vi "Impulse Response Function.vi"(1 "Signal Y Response":dbl[](array[numeric]) format="%0.2f", 2 "Signal X Stimulus":dbl[](array[numeric]) format="%0.2f") -> (0 "Impulse Response":dbl[](array[numeric]) format="%0.2f")   [LabVIEW 2020, in "NI_AALPro.lvlib"]
doc: "Computes the impulse response of a network based on time-domain signals Signal X Stimulus and Signal Y Response. The impulse response is in the time domain, so you do not need to convert time units to frequency units. The impulse response is the inverse transform of the transfer function.\n\nThe VI computes Impulse Response as\n Inverse Real FFT [ Sxy(f) / Sxx(f) ]\n\nSignal X Stimulus is a time-domain signal, usually the network stimulus.\n\nSignal Y Response is a time-domain signal, usually the network response.\n\nImpulse Response is the impulse response function versus time. This parameter is unitless."
uses:
  <vilib>/Analysis/NI_AALPro.lvlib
  <vilib>/Analysis/2dsp.llb/Cross Power (DBL).vi
panel:
  # "Impulse Response Function"
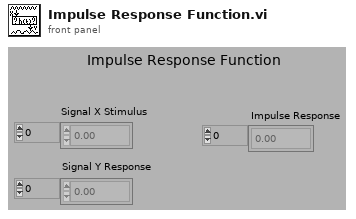
[diagram p1: front panel]
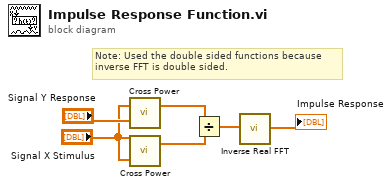
[diagram p0: block diagram]
diagram:
  # "Note: Used the double sided functions because\ninverse FFT is double sided."
  n1 = call-poly <vilib>:"Cross Power.vi"("Y"="Signal Y Response", "X"="Signal X Stimulus") -> ("Sxy"=w3:cdb[])  [unwired: 1 out]
  n2 = call-poly <vilib>:"Cross Power.vi"("Y"="Signal X Stimulus", "X"="Signal X Stimulus") -> ("Sxy"=w2:cdb[])  [unwired: 1 out]
  n3 = Divide(x=w3, y=w2) -> (x/y=w1:cdb[])
  n4 = call <vilib>:"Inverse Real FFT.vi"("FFT {X}"=w1) -> ("X"=→"Impulse Response":dbl[])  [unwired: 9 in, 1 out]
